vi "Launch Tasks.vi"(8 "error in (no error)":errorcluster, 11 "Study Actor in":refnum<class "Study Actor.lvclass">) -> (0 "error out":errorcluster, 3 "Study Actor out":refnum<class "Study Actor.lvclass">)   [LabVIEW 2023, in "Study Actor.lvlib" / "Study Actor.lvclass"]
uses:
  Study Actor.lvclass
  Study Actor.lvclass/Study Actor.ctl
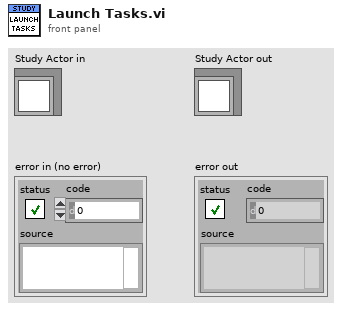
[diagram p1: front panel]
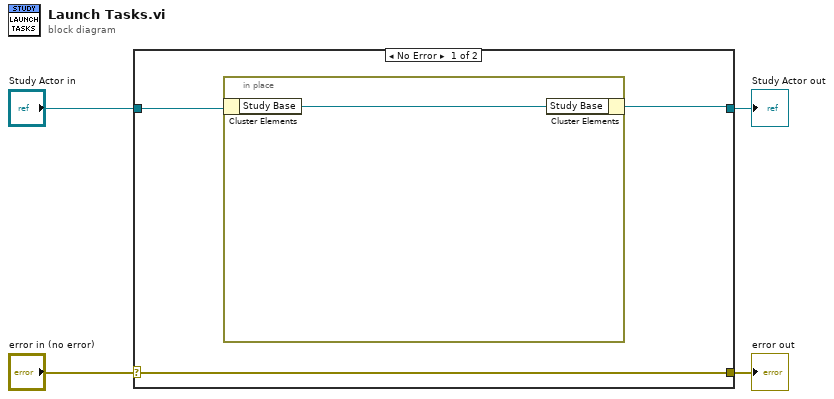
[diagram p0: block diagram]
diagram:
  n1 = case shown="No Error" "error in (no error)" {
    selector: "error in (no error)" -> [w7 w10]
    tunnel: [w7 w10] -> w3
    tunnel: [w5 w9] -> w1
    tunnel: "Study Actor in" -> [w6 w9]
    frame No Error {
      n2 = in-place {
        n3 = in-place-cluster #1(w6) -> ("Study Base"=w8:refnum<class "Study Base.lvclass">)
        n4 = in-place-cluster #1("Study Base"=w8) -> (w5:refnum<class "Study Actor.lvclass">)
      }
    }
    frame Error {
    }
  }
  "error out" <- w3
  "Study Actor out" <- w1
